vi "Test TX to Multi RX.vi"() -> ()   [LabVIEW 2021]
uses:
  typedef/CAN Port Configuration.ctl
  typedef/CAN Mode.ctl
  typedef/FD Config.ctl
  Channels/ChannelCommon/typedef/Datatype CAN.ctl
  CAN_Logic.lvclass/CAN_Logic.ctl
  Utilities/Decode Tags.vi
  Utilities/Check Packet Length.vi
  Utilities/TX Timeout.vi
  <vilib>/Utility/error.llb/Clear Errors.vi
  CIFUtilities/CIFClocks/Time Conversion/LabVIEW Time to UTC Time.vi
  Utilities/Encode Tags.vi
  typedef/Error Global.vi
  <vilib>/xnet/xnet.llb/XNET Write.vi
  <vilib>/xnet/xnet.llb/XNET Write (Frame CAN).vi
  <vilib>/xnet/xnet.llb/XNET Read.vi
  <vilib>/xnet/xnet.llb/XNET Read (Frame CAN).vi
  CAN_Logic.lvclass
  Channels/ChannelCommon/ChannelCommon.lvlib
panel:
  out "Pass":bool
  out "Local Subordinate":T1[](array[typedef]) {"Tags" format="%.0x"; "payload" format="%x"; "identifier" format="%x"}
  out "Local CAN":T1[](array[typedef]) {"Tags" format="%.0x"; "payload" format="%x"; "identifier" format="%x"}
  out "Remote CAN":T1[](array[typedef]) {"Tags" format="%.0x"; "payload" format="%x"; "identifier" format="%x"}
  out "error out":errorcluster
  in  "CAN Data":T1[](array[typedef])=[{"payload"=[0, 0, 0, 0, 0, 0, 0, 51], "identifier"=1, "Tags"=0, "Timestamp"=0}, {"payload"=[0, 0, 0, 0, 0, 0, 0, 36], "identifier"=2, "Tags"=0, "Timestamp"=0}] {"Tags" format="%.0x"; "payload" format="%x"; "identifier" format="%x"}
  in  "Port Configuration":T2={"Mode"=enum."CAN FD", "Baud Rate"=500000, "Temination On"=TRUE, "Subordinate"=FALSE, "Echo TX"=FALSE, "FD Config"={"FD Baud Rate"=2000000, "ISO Mode"=TRUE, "BRS Enabled"=TRUE}} {"FD Config"."FD Baud Rate" format="%.0p"; "Baud Rate" format="%.0p"}
  in  "RX Initerface":string="CAN2"
  in  "TX Interface":string="CAN1"
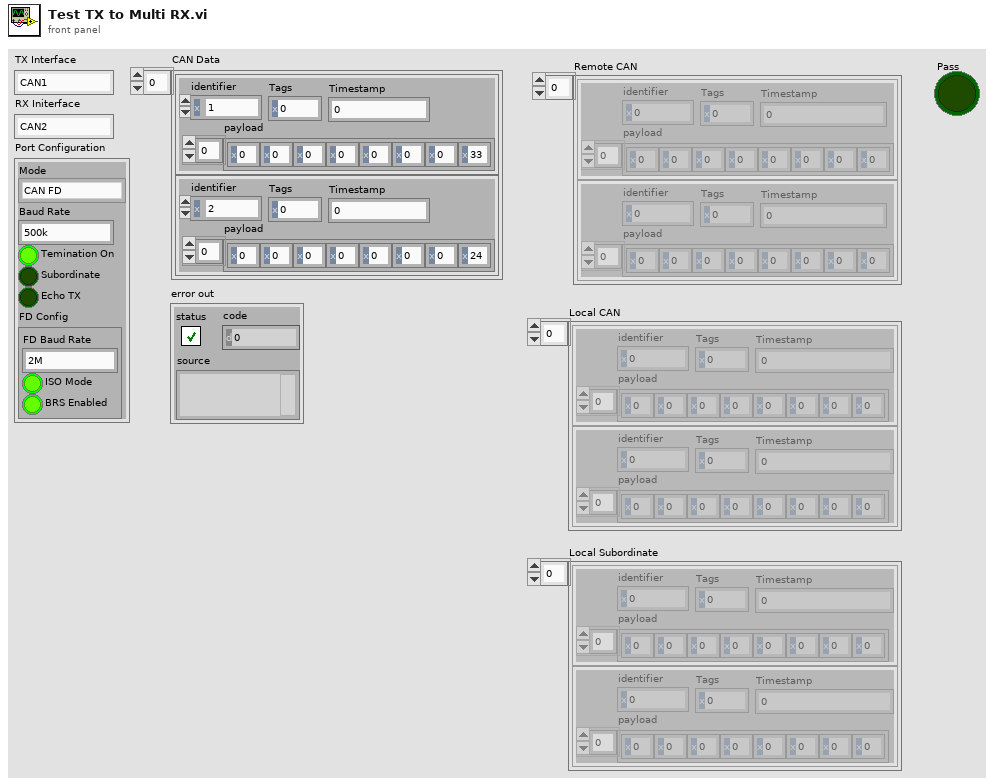
[diagram p1: front panel]
types:
  T1 = typedef "ChannelCommon.lvlib/Datatype CAN.ctl" = cluster{"payload":u8[], "identifier":u32, "Tags":u8, "Timestamp":u64}
  T2 = typedef "CAN_Logic.lvclass/CAN Port Configuration.ctl" = cluster{"Mode":T3, "Baud Rate":u64, "Temination On":bool, "Subordinate":bool, "Echo TX":bool, "FD Config":T4}
  T3 = typedef "CAN_Logic.lvclass/CAN Mode.ctl" = enum16{"CAN 2.0", "CAN FD"}
  T4 = typedef "CAN_Logic.lvclass/FD Config.ctl" = cluster{"FD Baud Rate":u64, "ISO Mode":bool, "BRS Enabled":bool}
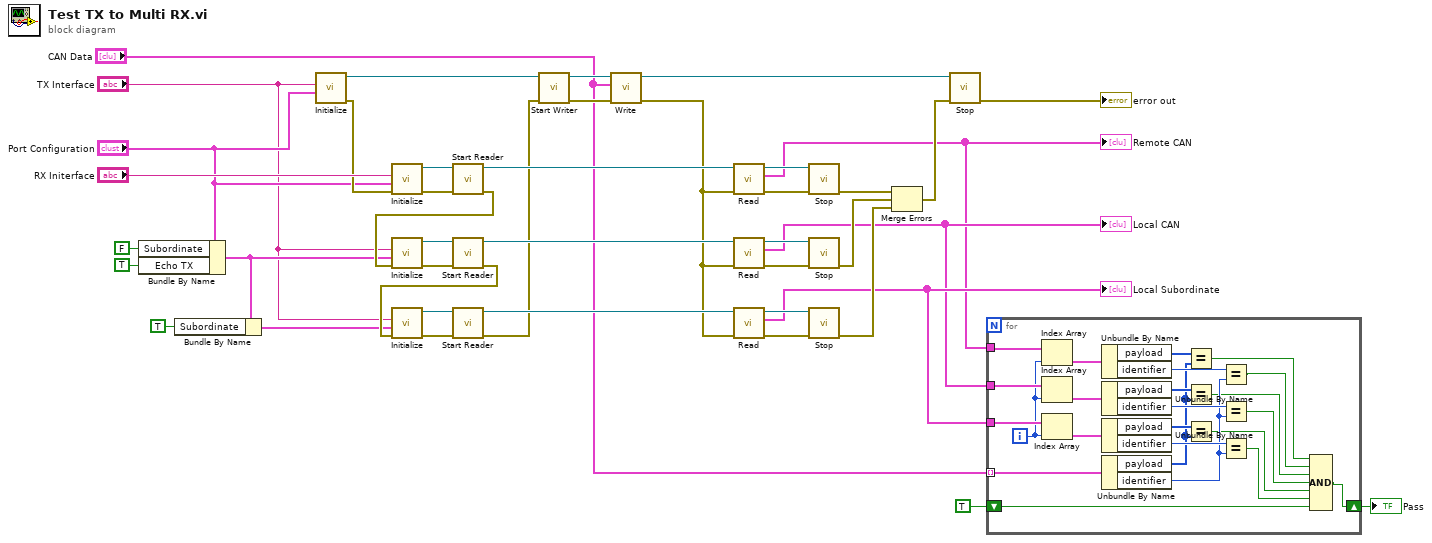
[diagram p0: block diagram]
diagram:
  n1 = Bundle By Name(cluster="Port Configuration", "Subordinate"=FALSE, "Echo TX"=TRUE) -> (w13:T2)
  n2 = Bundle By Name(cluster=w13, "Subordinate"=TRUE) -> (w12:T2)
  n3 = call "Initialize.vi"("Port Configuration"="Port Configuration", "Interface"="TX Interface") -> ("error out"=w42:errorcluster, "CAN_Logic out"=w41:refnum<class "CAN_Logic.lvclass">)  [unwired: 8 in]
  n4 = call "Initialize.vi"("error in (no error)"=w42, "Port Configuration"="Port Configuration", "Interface"="RX Initerface") -> ("error out"=w39:errorcluster, "CAN_Logic out"=w40:refnum<class "CAN_Logic.lvclass">)  [unwired: 7 in]
  n5 = call "Start Reader.vi"("error in (no error)"=w39, "CAN_Logic in"=w40) -> ("error out"=w26:errorcluster, "CAN_Logic out"=w36:refnum<class "CAN_Logic.lvclass">)  [unwired: 8 in]
  n6 = call "Initialize.vi"("error in (no error)"=w26, "Port Configuration"=w13, "Interface"="TX Interface") -> ("error out"=w28:errorcluster, "CAN_Logic out"=w27:refnum<class "CAN_Logic.lvclass">)  [unwired: 7 in]
  n7 = call "Start Reader.vi"("error in (no error)"=w28, "CAN_Logic in"=w27) -> ("error out"=w17:errorcluster, "CAN_Logic out"=w29:refnum<class "CAN_Logic.lvclass">)  [unwired: 8 in]
  n8 = call "Initialize.vi"("error in (no error)"=w17, "Port Configuration"=w12, "Interface"="TX Interface") -> ("error out"=w21:errorcluster, "CAN_Logic out"=w22:refnum<class "CAN_Logic.lvclass">)  [unwired: 7 in]
  n9 = call "Start Reader.vi"("error in (no error)"=w21, "CAN_Logic in"=w22) -> ("error out"=w16:errorcluster, "CAN_Logic out"=w20:refnum<class "CAN_Logic.lvclass">)  [unwired: 8 in]
  n10 = call "Start Writer.vi"("error in (no error)"=w16, "CAN_Logic in"=w41) -> ("error out"=w37:errorcluster, "CAN_Logic out"=w38:refnum<class "CAN_Logic.lvclass">)  [unwired: 8 in]
  n11 = call "Write.vi"("error in (no error)"=w37, "CAN Data"="CAN Data", "CAN_Logic in"=w38) -> ("error out"=w15:errorcluster, "CAN_Logic out"=w33:refnum<class "CAN_Logic.lvclass">)  [unwired: 7 in]
  n12 = call "Read.vi"("error in (no error)"=w15, "CAN_Logic in"=w36) -> ("error out"=w34:errorcluster, "CAN Data"=w3:T1[], "CAN_Logic out"=w35:refnum<class "CAN_Logic.lvclass">)  [unwired: 6 in, 1 out]
  "Remote CAN" <- w3
  n13 = call "Read.vi"("error in (no error)"=w15, "CAN_Logic in"=w29) -> ("error out"=w31:errorcluster, "CAN Data"=w4:T1[], "CAN_Logic out"=w30:refnum<class "CAN_Logic.lvclass">)  [unwired: 6 in, 1 out]
  "Local CAN" <- w4
  n14 = call "Read.vi"("error in (no error)"=w15, "CAN_Logic in"=w20) -> ("error out"=w18:errorcluster, "CAN Data"=w5:T1[], "CAN_Logic out"=w19:refnum<class "CAN_Logic.lvclass">)  [unwired: 6 in, 1 out]
  "Local Subordinate" <- w5
  n15 = call "Stop.vi"("error in (no error)"=w34, "CAN_Logic in"=w35) -> ("error out"=w10:errorcluster)  [unwired: 8 in, 1 out]
  n16 = call "Stop.vi"("error in (no error)"=w31, "CAN_Logic in"=w30) -> ("error out"=w9:errorcluster)  [unwired: 8 in, 1 out]
  n17 = call "Stop.vi"("error in (no error)"=w18, "CAN_Logic in"=w19) -> ("error out"=w8:errorcluster)  [unwired: 8 in, 1 out]
  n18 = Merge Errors(w10, w9, w8) -> (w7:errorcluster)
  n19 = call "Stop.vi"("error in (no error)"=w7, "CAN_Logic in"=w33) -> ("error out"=→"error out":errorcluster)  [unwired: 8 in, 1 out]
  n20 = for {
    tunnel: "CAN Data" -> [w67] mode=indexing
    tunnel: w5 -> [w48]
    tunnel: w4 -> [w47]
    tunnel: w3 -> [w50]
    shift-right: [w51] -> w1
    shift-left: TRUE -> [w52]
    i -> [w44]
    n21 = Index Array(array=w50, index=w44) -> (element=w49:T1)
    n22 = Index Array(array=w47, index=w44) -> (element=w46:T1)
    n23 = Index Array(array=w48, index=w44) -> (element=w45:T1)
    n24 = Unbundle By Name(w49) -> ("payload"=w66:u8[], "identifier"=w65:u32)
    n25 = Unbundle By Name(w46) -> ("payload"=w63:u8[], "identifier"=w64:u32)
    n26 = Unbundle By Name(w45) -> ("payload"=w62:u8[], "identifier"=w61:u32)
    n27 = Unbundle By Name(w67) -> ("payload"=w60:u8[], "identifier"=w59:u32)
    n28 = Equal?(x=w66, y=w60) -> (x = y?=w58:bool)
    n29 = Equal?(x=w63, y=w60) -> (x = y?=w56:bool)
    n30 = Equal?(x=w62, y=w60) -> (x = y?=w54:bool)
    n31 = Equal?(x=w65, y=w59) -> (x = y?=w57:bool)
    n32 = Equal?(x=w64, y=w59) -> (x = y?=w55:bool)
    n33 = Equal?(x=w61, y=w59) -> (x = y?=w53:bool)
    n34 = Compound Arithmetic op=AND(w58, w57, w56, w55, w54, w53, w52) -> (w51:bool)
  }
  "Pass" <- w1
